vi "GetDLLPath.vi"(8 "Error In":errorcluster) -> (0 "Error Out":errorcluster, 1 "Bit System":T1, 2 "SPC Folder Path":path=path "C:/Program Files (x86)/BH/SPCM/DLL", 3 "DLL Path":path)   [LabVIEW 2023]
doc: "All wrapper VIs for spcmdll calls need the filepath to the dll. This VI provides this path according to the operation systems bitness and the LabVIEW bitness.\n\ninfo@becker-hickl.com"
panel:
  out "CMD Output":string="This is the output from Windows Command Prompt. "
  out "String before \"-bit\"":string="This the same output, but only the portion before \"-bit\" in the original output. "
  out "32/64 subset":string="Substring containing \"32\" or \"64\""
  # "Overview: This VI parses the string output of the System Exec VI to determine if the Windows Environment is 32-bit or 64-bit.\nRequirement: LabVIEW 2012 or compatible\nInstructions:\n1. Run the VI.\n2. Check the lights to see if it is 32/64 bit OS"
  # "This VI was checked by National Instruments and was verified. Further, this VI was afterwards\nchanged to determine the correct DLL path for further use.\n\ninfo@becker-hickl.com"
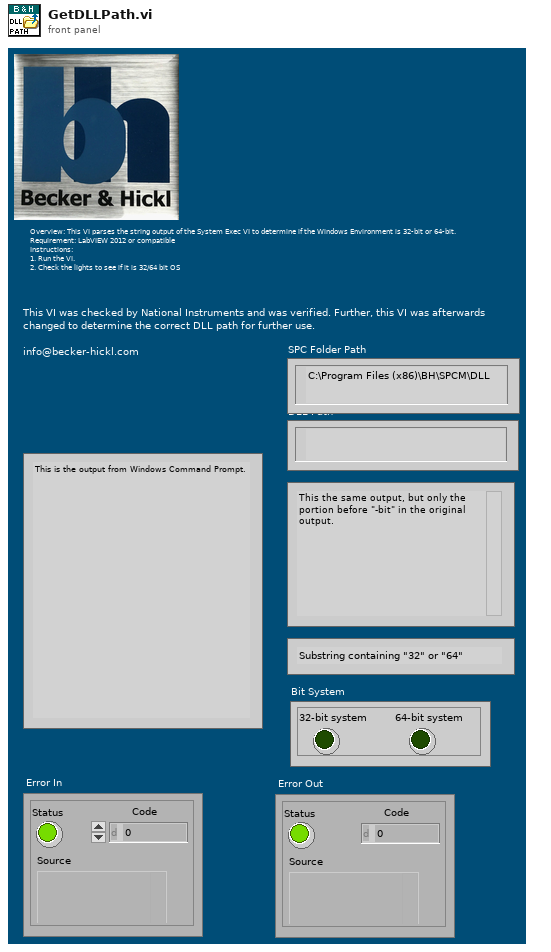
[diagram p1: front panel]
types:
  T1 = cluster{"32-bit system":bool, "64-bit system":bool}
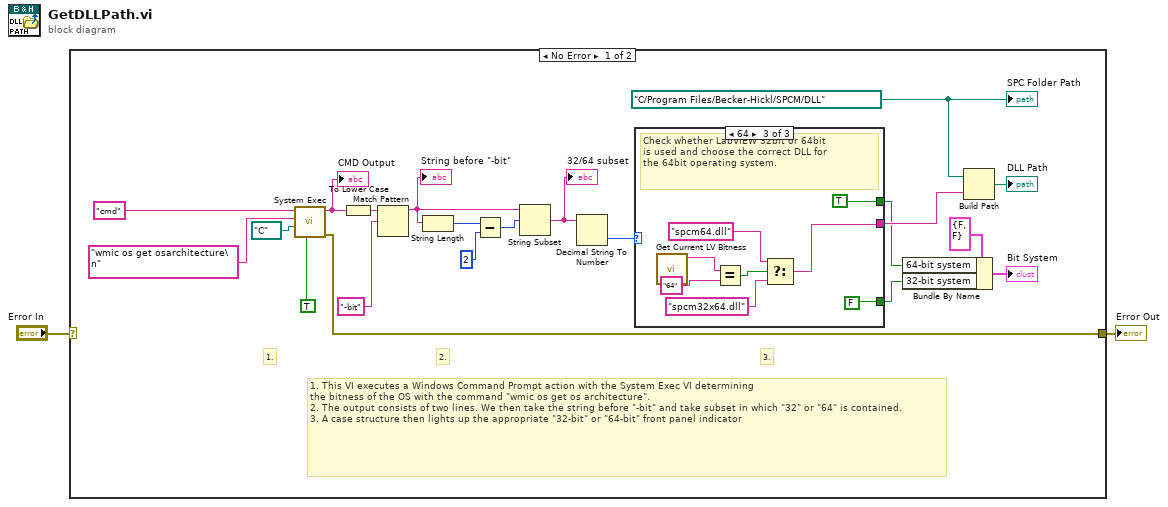
[diagram p0: block diagram]
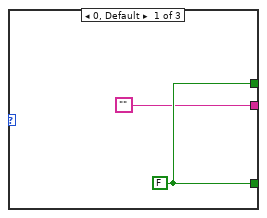
[diagram p2: hidden frame]
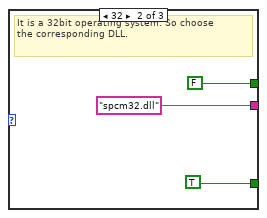
[diagram p3: hidden frame]
diagram:
  n1 = case shown="No Error" "Error In" {
    selector: "Error In" -> [_ w37]
    tunnel: [w8 w37] -> w1
    frame No Error {
      w12 = path "C:/Program Files/Becker-Hickl/SPCM/DLL"
      # "1. This VI executes a Windows Command Prompt action with the System Exec VI determining \nthe bitness of the OS with the command \"wmic os get os architecture\".  \n2. The output consists of two lines. We then take the string before \"-bit\" and take subset in which \"32\" or \"64\" is contained.  \n3. A case structure then lights up the appropriate \"32-bit\" or \"64-bit\" front panel indicator"
      # "3."
      # "2."
      # "1."
      n2 = call <vilib>:"System Exec.vi"("run minimized? (F)"=TRUE, "working directory"=path "C:/", "standard input"="wmic os get osarchitecture\n", "command line"="cmd") -> ("error out"=w8:errorcluster, "standard output"=w13:string)  [unwired: 4 in, 2 out]
      "CMD Output" <- w13
      n3 = To Lower Case(string=w13) -> (all lower case string=w9:string)
      n4 = Match Pattern(string=w9, regular expression="-bit") -> (before substring=w14:string)  [unwired: 1 in, 3 out]
      "String before \"-bit\"" <- w14
      n5 = String Length(string=w14) -> (length=w18:i32)
      n6 = Subtract(x=w18, y=2) -> (x-y=w16:i32)
      n7 = String Subset(string=w14, offset (0)=w16) -> (substring=w15:string)  [unwired: 1 in]
      "32/64 subset" <- w15
      n8 = Decimal String To Number(string=w15) -> (number=w3:i32)  [unwired: 2 in, 1 out]
      n9 = case shown="64" w3 {
        tunnel: [w25 FALSE TRUE] -> w6
        tunnel: [w25 TRUE FALSE] -> w5
        tunnel: ["" "spcm32.dll" w31] -> w11
        frame 0, Default {
          w25 = FALSE
        }
        frame 32 {
          # "It is a 32bit operating system. So choose\nthe corresponding DLL."
        }
        frame 64 {
          # "Check whether LabVIEW 32bit or 64bit\nis used and choose the correct DLL for \nthe 64bit operating system."
          n10 = call <vilib>:"Get Current LV Bitness.vi"() -> ("bitness"=w34:string)  [unwired: 11 in]
          n11 = Equal?(x=w34, y="64") -> (x = y?=w32:bool)
          n12 = Select(t="spcm64.dll", s=w32, f="spcm32x64.dll") -> (s? t:f=w31:string)
        }
      }
      n13 = Bundle By Name(cluster=T1 {"32-bit system"=FALSE, "64-bit system"=FALSE} ("Bit System 2"), "64-bit system"=w6, "32-bit system"=w5) -> (→"Bit System":T1)
      n14 = Build Path(base path=w12, name or relative path=w11) -> (appended path=→"DLL Path":path)
      "SPC Folder Path" <- w12
    }
    frame Error {
    }
  }
  "Error Out" <- w1
